vi "Sanitize list.vi"(11 "List":string[](array[string])) -> (3 "sanitized list":string[](array[string]))   [LabVIEW 2021, in "Autocomplete Textbox.lvlib"]
uses:
  Autocomplete Textbox.lvlib
  <userlib>/_OpenG.lib/array/array.llb/Remove Duplicates from 1D Array (String)__ogtk.vi
  <userlib>/_OpenG.lib/array/array.llb/Filter 1D Array with Scalar (String)__ogtk.vi
  <userlib>/_OpenG.lib/array/array.llb/openg_array.lvlib
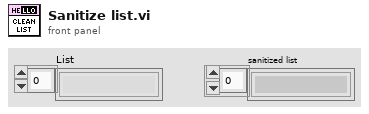
[diagram p1: front panel]
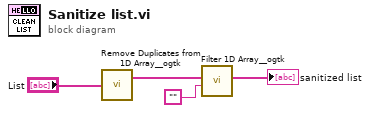
[diagram p0: block diagram]
diagram:
  n1 = call-poly <userlib>:"Remove Duplicates from 1D Array__ogtk.vi"("Input Array"="List") -> ("Output Array"=w4:string[])  [unwired: 1 out]
  n2 = call-poly <userlib>:"Filter 1D Array__ogtk.vi"("items to filter"="", "array"=w4) -> ("filtered array"=→"sanitized list":string[])  [unwired: 4 in, 1 out]
